vi "create-wfm-dvr.vi"(8 "error in (no error)":errorcluster) -> (0 "error out":errorcluster, 3 "wfm dvr":refnum<data-value>)   [LabVIEW 2024]
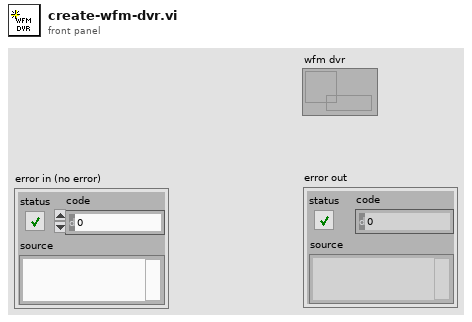
[diagram p1: front panel]
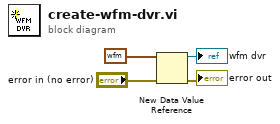
[diagram p0: block diagram]
diagram:
  n1 = New Data Value Reference(data value=waveform(dbl) {"t0"=timestamp(0 s since 1904-01-01), "dt"=1.0, "Y"=[]} ("Waveform"), error in="error in (no error)") -> (data value reference=→"wfm dvr":refnum<data-value>, error out=→"error out":errorcluster)
